vi "Device Property - Get SV Update Rate.vi"(8 "error in (no error)":errorcluster, 11 "Device Ref in":T1 format="%.0x") -> (0 "error out":errorcluster, 2 "Update Rate (ms)":dbl format="%.2f", 3 "Device Ref out":T1 format="%.0x")   [LabVIEW 2017]
uses:
  <vilib>/NI Veristand/Custom Device API/Custom Device Item Ref.ctl
  SV Global.vi
  <vilib>/NI Veristand/Custom Device API/Get Item Property (Double).vi
  <vilib>/NI VeriStand/Custom Device API/Custom Device API.lvlib
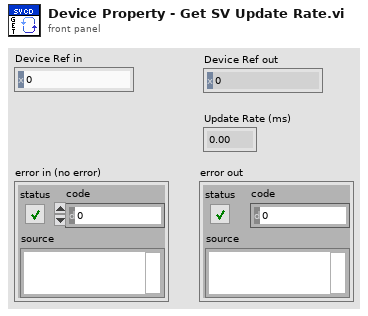
[diagram p1: front panel]
types:
  T1 = typedef "Custom Device API.lvlib/Custom Device Item Ref.ctl" = u64
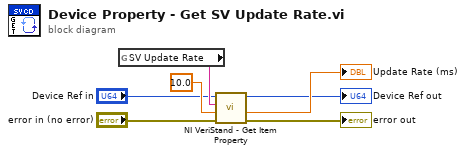
[diagram p0: block diagram]
diagram:
  n1 = global read "SV Global.vi" "SV Update Rate"() -> (w7:string)
  n2 = call-poly <vilib>:"NI VeriStand - Get Item Property.vi"("error in (no error)"="error in (no error)", "Default Value"=10.0, "Property Name"=w7, "Item Ref in"="Device Ref in") -> ("error out"=→"error out":errorcluster, "Value"=→"Update Rate (ms)":dbl, "Item Ref out"=→"Device Ref out":T1)  [unwired: 4 in, 1 out]
